vi "ex4.vi"() -> ()   [LabVIEW 2022 SP3]
panel:
  out "Output string":string
  in  "input":string
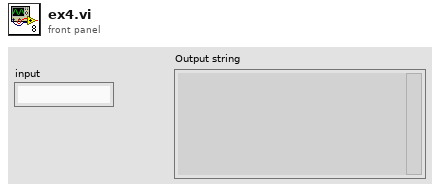
[diagram p1: front panel]
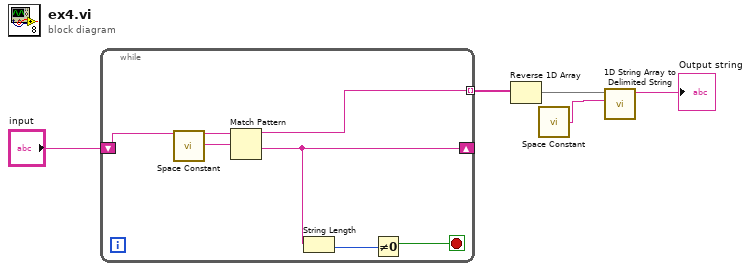
[diagram p0: block diagram]
diagram:
  n1 = while {
    shift-right: [w7] -> _
    shift-left: "input" -> [w9]
    tunnel: [w6] -> w1 mode=indexing
    stop <- w11 stop-if-true
    n2 = call <vilib>:"Space Constant.vi"() -> ("String"=w8:string)
    n3 = Match Pattern(string=w9, regular expression=w8) -> (before substring=w6:string, after substring=w7:string)  [unwired: 1 in, 2 out]
    n4 = String Length(string=w7) -> (length=w10:i32)
    n5 = Not Equal To 0?(x=w10) -> (x != 0?=w11:bool)
  }
  n6 = Reverse 1D Array(array=w1) -> (reversed array=w5:string[])
  n7 = call <vilib>:"Space Constant.vi"() -> ("String"=w4:string)
  n8 = call <vilib>:"1D String Array to Delimited String.vi"("delimiter"=w4, "string array"=w5) -> ("delimited string"=→"Output string":string)  [unwired: 9 in]
